vi "Read Write Script.vi"(6 "chip select (0)":u32, 8 "error in (no error)":errorcluster, 9 "Write Data":u8[](array[numeric]), 10 "delay in milliseconds (0)":u8, 11 "spi script reference in":T1) -> (0 "error out":errorcluster, 1 "script read index":u32, 3 "spi script reference out":T1)   [LabVIEW 2013]
doc: "To be used in a USB-8451 script:\n\nPerforms a read-write operation on the channel with the given chip select pin. Write data is an array of bytes to send. The returned script read index can be used later in the same script to obtain the returned data, if any. The optional delay increases the time between toggling CS and sending the data."
uses:
  <vilib>/ni845x/ni845x.llb/ni845xSpiScriptControl.ctl
  <vilib>/ni845x/ni845x.llb/NI-845x SPI Script Ms Delay.vi
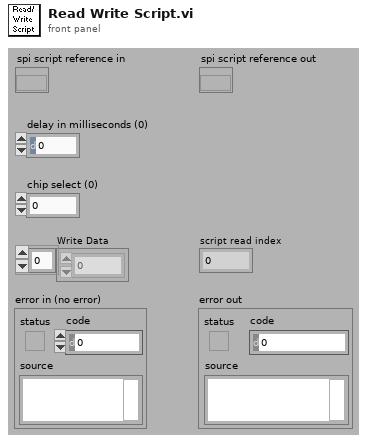
[diagram p1: front panel]
types:
  T1 = typedef "ni845xSpiScriptControl.ctl" = refnum<k20>
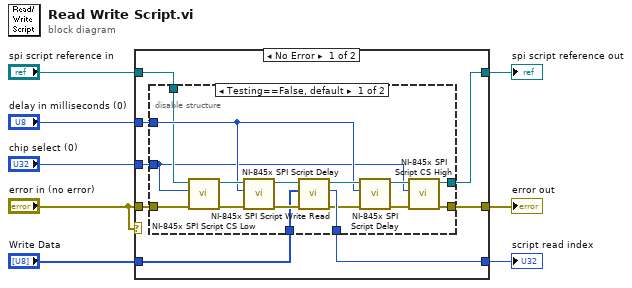
[diagram p0: block diagram]
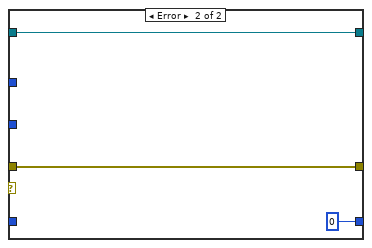
[diagram p3: hidden frame]
diagram:
  n1 = case shown="No Error" "error in (no error)" {
    tunnel: [w16 u32 0 ("script read index")] -> w8
    tunnel: [w15 w35] -> w7
    tunnel: [w14 w37] -> w6
    tunnel: "Write Data" -> [w13 _]
    tunnel: "delay in milliseconds (0)" -> [w12 _]
    tunnel: "error in (no error)" -> [w11 w37]
    tunnel: "spi script reference in" -> [w10 w35]
    tunnel: "chip select (0)" -> [w9 _]
    frame No Error {
      n2 = disable-structure shown="Testing==False, default" {
        disable-tunnel: [w32 _] -> w16
        disable-tunnel: [w23 w33] -> w15
        disable-tunnel: [w22 w34] -> w14
        disable-tunnel: w13 -> [w21 _]
        disable-tunnel: w12 -> [w20 _]
        disable-tunnel: w11 -> [w19 w34]
        disable-tunnel: w10 -> [w18 w33]
        disable-tunnel: w9 -> [w17 _]
        frame condition #0 (active) {
          n3 = call <vilib>:"NI-845x SPI Script CS Low.vi"("error in (no error)"=w19, "chip select (0)"=w17, "spi script reference in"=w18) -> ("error out"=w26:errorcluster, "spi script reference out"=w27:T1)  [unwired: 7 in]
          n4 = call-poly <vilib>:"NI-845x SPI Script Delay.vi"("error in (no error)"=w26, "delay in milliseconds (0)"=w20, "spi script reference in"=w27) -> ("error out"=w24:errorcluster, "spi script reference out"=w25:T1)  [unwired: 7 in]
          n5 = call <vilib>:"NI-845x SPI Script Write Read.vi"("error in (no error)"=w24, "write data"=w21, "spi script reference in"=w25) -> ("error out"=w31:errorcluster, "script read index"=w32:u32, "spi script reference out"=w30:T1)  [unwired: 6 in]
          n6 = call-poly <vilib>:"NI-845x SPI Script Delay.vi"("error in (no error)"=w31, "delay in milliseconds (0)"=w20, "spi script reference in"=w30) -> ("error out"=w28:errorcluster, "spi script reference out"=w29:T1)  [unwired: 7 in]
          n7 = call <vilib>:"NI-845x SPI Script CS High.vi"("error in (no error)"=w28, "chip select (0)"=w17, "spi script reference in"=w29) -> ("error out"=w22:errorcluster, "spi script reference out"=w23:T1)  [unwired: 7 in]
        }
        frame condition #1 {
        }
      }
    }
    frame Error {
    }
  }
  "script read index" <- w8
  "spi script reference out" <- w7
  "error out" <- w6
